vi "Optimal Control Design.vi"() -> ()   [LabVIEW 2018]
uses:
  <vilib>/addons/Control Design/_Model Construction/Model Creation.llb/Model Creation SubVI/cd_Create State Space Model.vi
  <vilib>/addons/Control Design/_Dynamic Analysis/Dynamic Analysis.llb/Dynamic Analysis subVI/cd_Pole-Zero Map (State-Space).vi
  <vilib>/addons/Control Design/_Utility/Model Viewer.llb/Model Viewer SubVI/cd_Draw State-Space Equation (SS).vi
  <vilib>/addons/Control Design/_State Feedback Control/State Feedback Control.llb/State Feedback Control SubVis/cd_Linear Quadratic Regulator.vi
  <vilib>/addons/Control Design/_Dynamic Analysis/NI_CD_Dynamic Analysis.lvlib
  <vilib>/addons/Control Design/_Model Construction/NI_LinSys_Model Creation.lvlib
  <vilib>/addons/Control Design/_Utility/NI_CD_Model Viewer.lvlib
  <vilib>/addons/Control Design/_State Feedback Control/NI_CD_State Feedback Control.lvlib
panel:
  out "Feedback Gain K":dbl[][](array[numeric])=[[-0.9999999999999947, 34.24877577354303, -1.2254222672198232, 3.0776350640206243]] format="%#_4g"
  in  "R":dbl[][](array[numeric])=[[1.0]]
  in  "Q":dbl[][](array[numeric])=[[1.0, 0.0, 0.0, 0.0], [0.0, 1.0, 0.0, 0.0], [0.0, 0.0, 1.0, 0.0], [0.0, 0.0, 0.0, 1.0]]
  out "Poles":cdb[](array[numeric])=[-16.174828889209856+0.0i, 16.168951670075447+0.0i, -0.004522780865591975+0.0i, 0.0+0.0i] caption="Open Loop Poles" format="%#_3g"
  out "Open Loop State-Space Model":picture
  in  "stop":bool
  # "Engineering Trainer Boards"
  # "Controls Board"
  # "Optimal Control Design"
  # "Optimal Control Design"
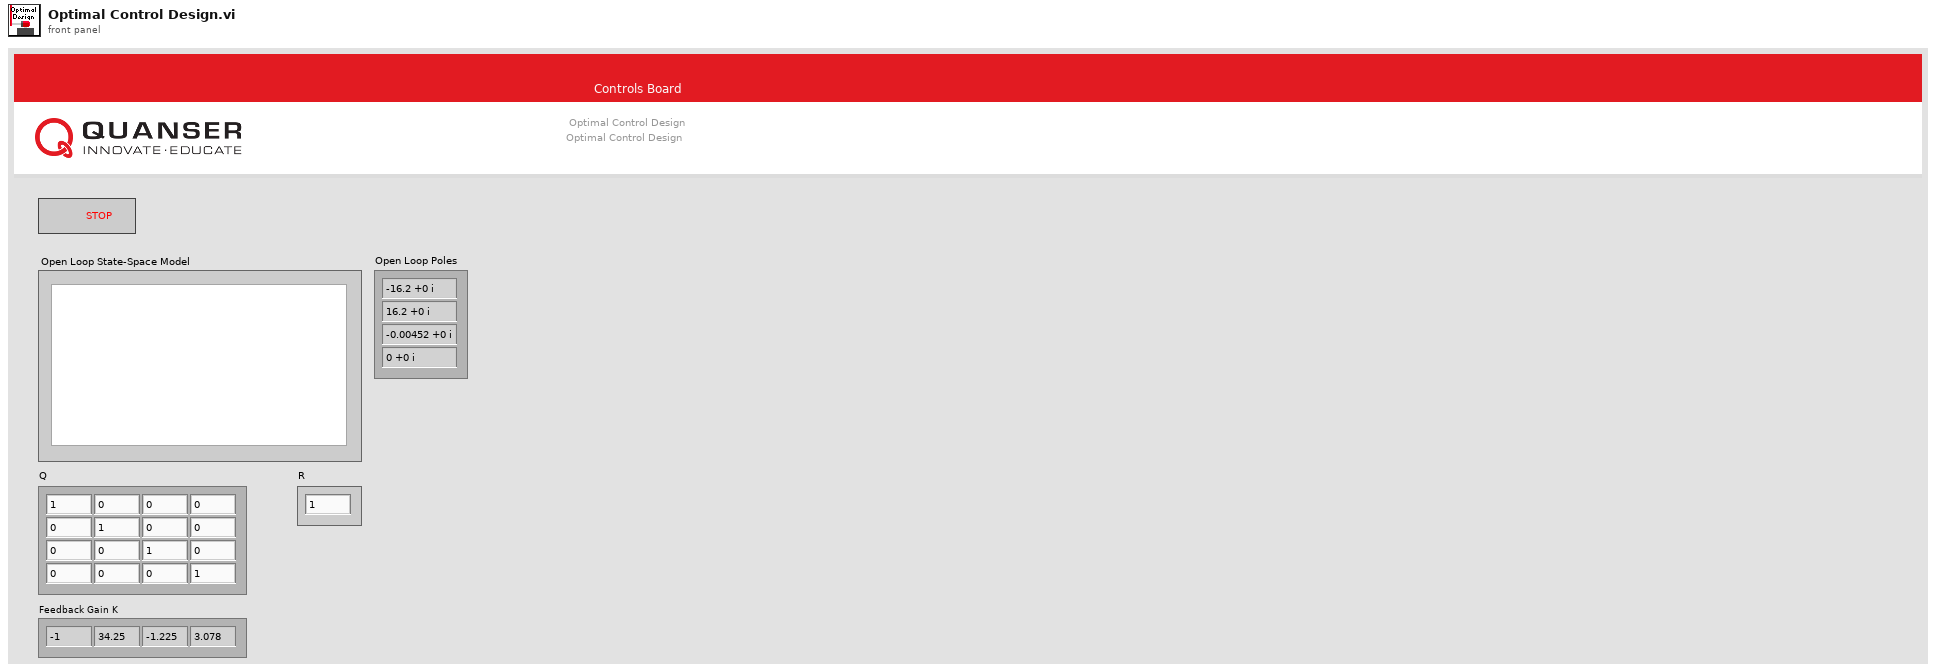
[diagram p1: front panel]
types:
  T1 = typedef "NI_LinSys_Model Typedefs.lvlib/CD State Space Model (MIMO).ctl" = cluster{"properties":T2, "A":dbl[][], "B":dbl[][], "C":dbl[][], "D":dbl[][], "StateNames":string[], "Transport Delay":dbl[][]}
  T2 = typedef "NI_LinSys_Model Typedefs.lvlib/CD General Elements.ctl" = cluster{"Model name":string, "Input names":string[], "Output names":string[], "Input Delays":dbl[], "Output Delays":dbl[], "Sampling Time":dbl, "Notes":string}
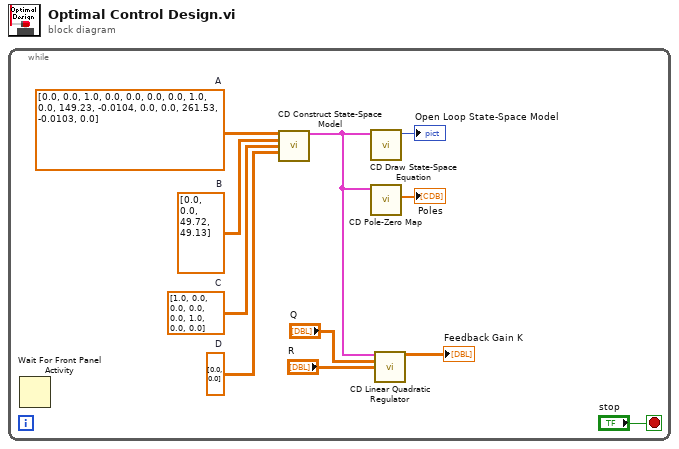
[diagram p0: block diagram]
diagram:
  n1 = while {
    stop <- "stop" stop-if-true
    w6 = dbl[][] [[0.0], [0.0]]  # D
    w7 = dbl[][] [[1.0, 0.0, 0.0, 0.0], [0.0, 1.0, 0.0, 0.0]]  # C
    w8 = dbl[][] [[0.0], [0.0], [49.72], [49.13]]  # B
    w9 = dbl[][] [[0.0, 0.0, 1.0, 0.0], [0.0, 0.0, 0.0, 1.0], [0.0, 149.23, -0.0104, 0.0], [0.0, 261.53, -0.0103, 0.0]]  # A
    n2 = Wait For Front Panel Activity() -> ()  [unwired: 3 in, 1 out]
    n3 = call-poly <vilib>:"CD Construct State-Space Model.vi"("A"=w9, "B"=w8, "C"=w7, "D"=w6) -> ("State-Space Model"=w4:T1)  [unwired: 10 in, 1 out]
    n4 = call-poly <vilib>:"CD Draw State-Space Equation.vi"("State-Space Model"=w4) -> ("Equation"=→"Open Loop State-Space Model":picture)  [unwired: 8 in, 2 out]
    n5 = call-poly <vilib>:"CD Pole-Zero Map.vi"("State-Space Model"=w4) -> ("Poles"=→"Poles":cdb[])  [unwired: 7 in, 3 out]
    n6 = call-poly <vilib>:"CD Linear Quadratic Regulator.vi"("State-Space Model"=w4, "Q"="Q", "R"="R") -> ("Optimal Gain (K)"=→"Feedback Gain K":dbl[][])  [unwired: 9 in, 3 out]
  }
